vi "Manual Assembly old.vi"() -> ()   [LabVIEW 2021]
uses:
  Classes/Routine/Routine Enum.ctl
  Classes/Routine/TypeOfHexaboard.ctl
  Classes/Assembly/Assembly Run.lvclass
  Classes/Workspace/Fixture Enum.ctl
  Classes/Controller/Controller.lvclass
  Classes/Workspace/Fixture.lvclass
  Classes/Routine/Routine.lvclass
panel:
  in  "Submit":bool
  out "Type of Hexaboard Confirmation":T1
  in  "Type of Component":T1
  in  "Update":bool
  in  "Stage":i32(listbox)=-1
  in  "Routine":T2=enum."Dispense on Plate"
  in  "Stop":bool
  in  "Remove":bool
  in  "Add":bool
  in  "Go":bool
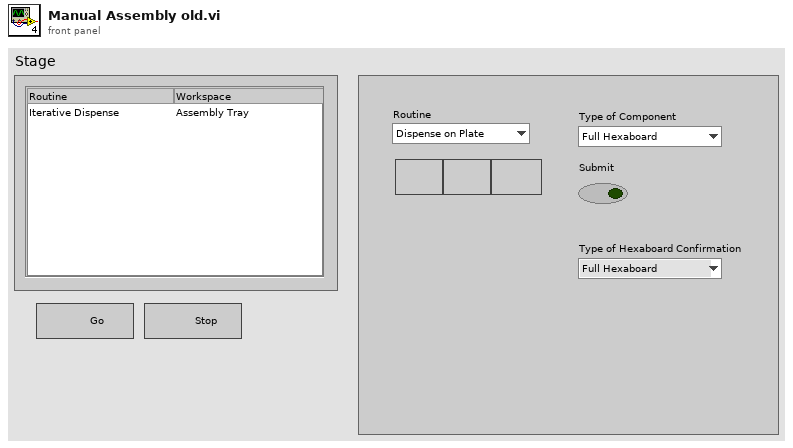
[diagram p1: front panel]
types:
  T1 = typedef "Routine.lvclass/TypeOfHexaboard.ctl" = enum16{"Full Hexaboard", "Right Partial PCB", "Right Partial Sensor", "Al Dummy Right Partial Sensor"}
  T2 = typedef "Routine.lvclass/Routine Enum.ctl" = enum16{"Primary Pick Up", "Secondary Pick Up", "Put Down All", "Secure Syringe", "Release Syringe", "Dispense on Plate", "Dispense on Sensor", "Pick Up All", "Put Down Secondary", "Dispense on Kapton"}
  T3 = typedef "Fixture.lvclass/Fixture Enum.ctl" = enum16{"Assembly Tray", "Syringe Space", "Component", "Pick Up Tool", "Current Position"}
  T4 = typedef "Controller.lvclass/Controllers.ctl" = cluster{"I-O.lvclass":refnum<class "I-O.lvclass">, "Gantry":refnum<k24>, "Dispenser":refnum<visa-resource-name>}
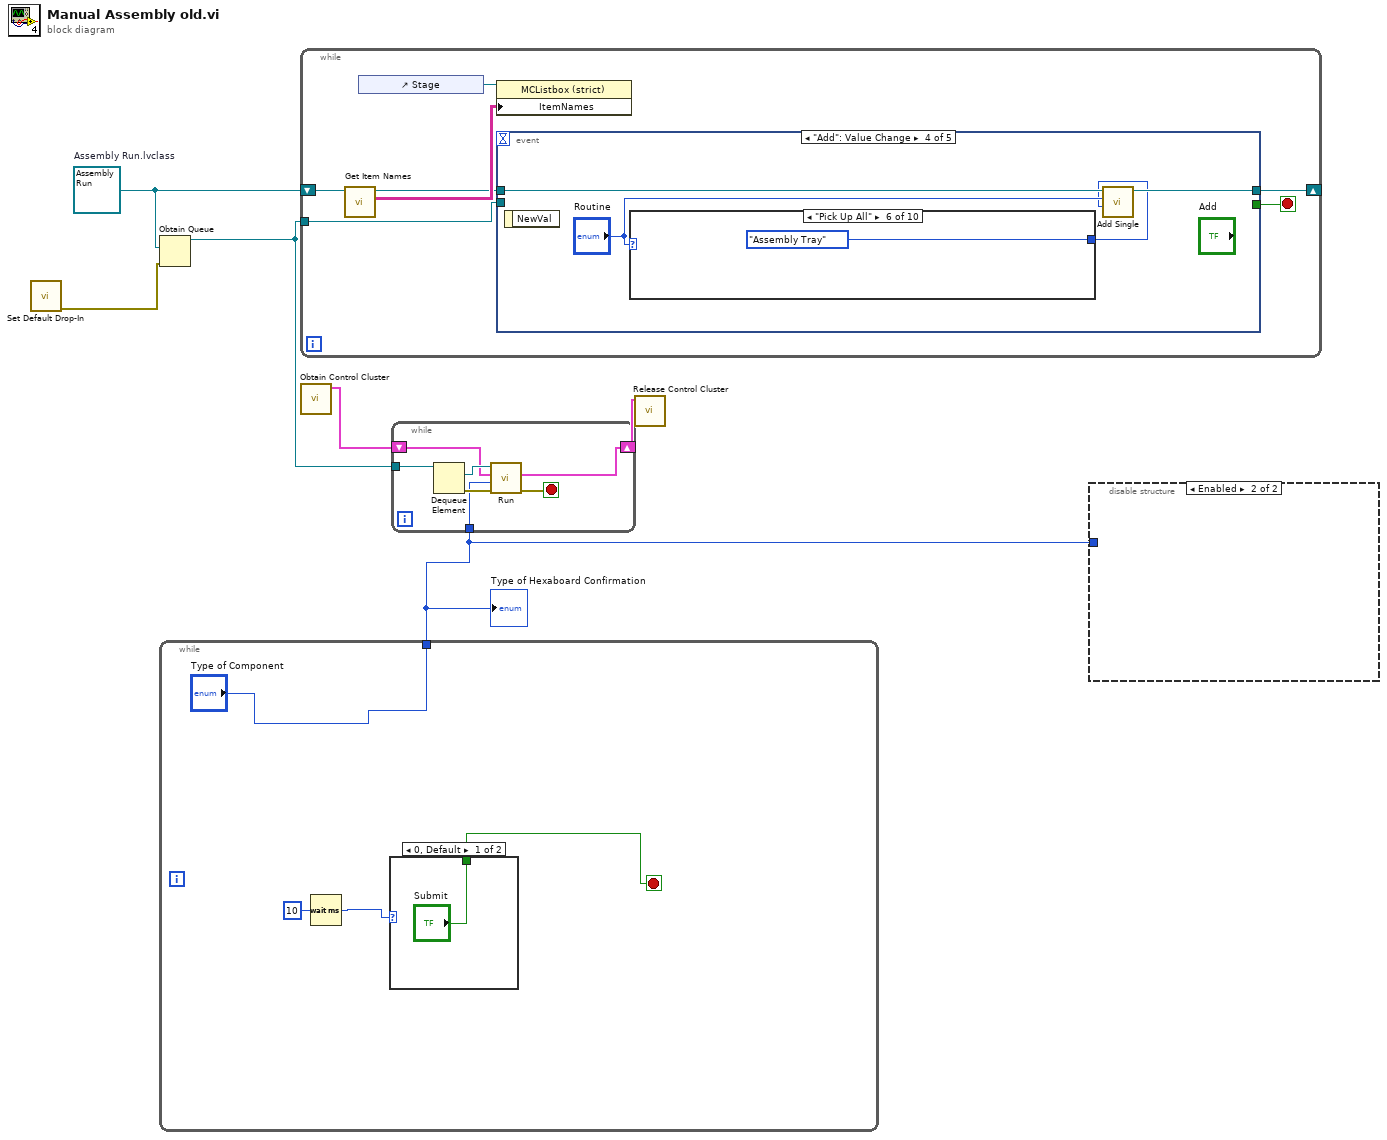
[diagram p0: block diagram]
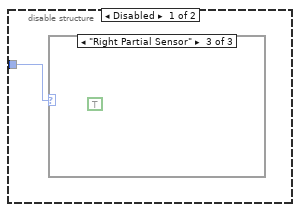
[diagram p2: hidden frame]
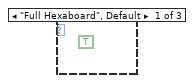
[diagram p3: hidden frame]
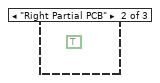
[diagram p4: hidden frame]
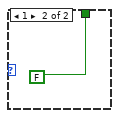
[diagram p5: hidden frame]
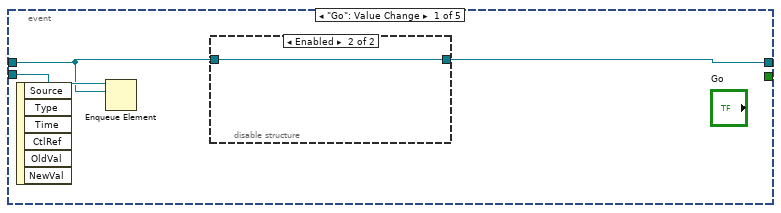
[diagram p6: hidden frame]
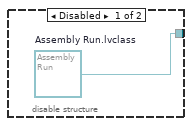
[diagram p7: hidden frame]
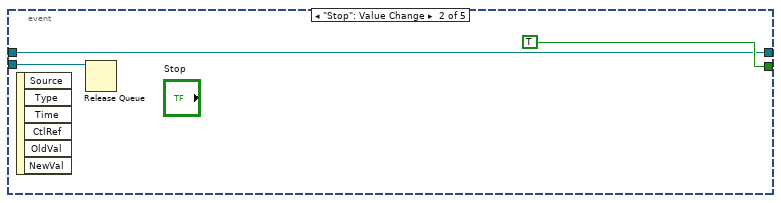
[diagram p8: hidden frame]
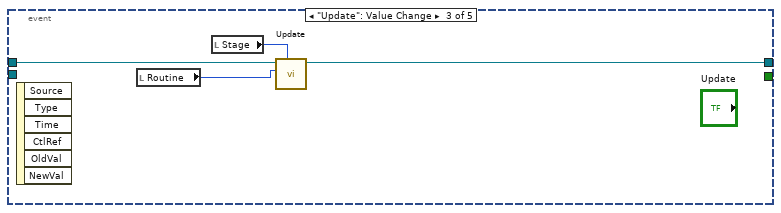
[diagram p9: hidden frame]
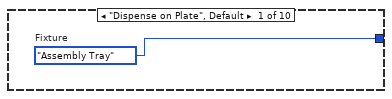
[diagram p10: hidden frame]
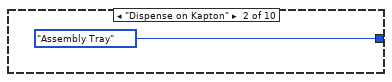
[diagram p11: hidden frame]
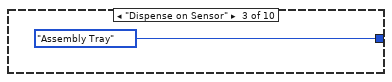
[diagram p12: hidden frame]
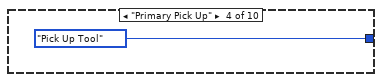
[diagram p13: hidden frame]
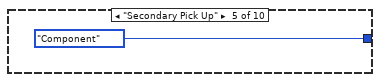
[diagram p14: hidden frame]
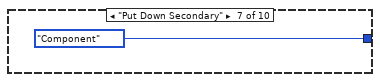
[diagram p15: hidden frame]
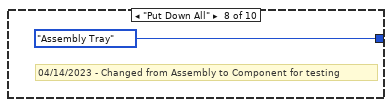
[diagram p16: hidden frame]
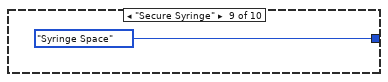
[diagram p17: hidden frame]
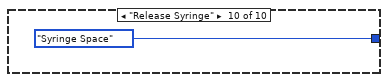
[diagram p18: hidden frame]
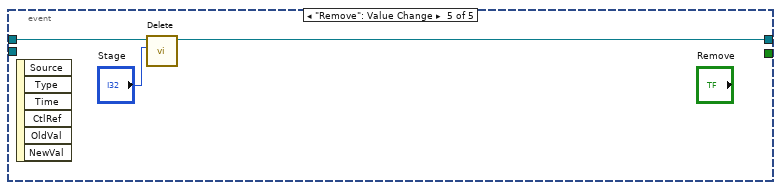
[diagram p19: hidden frame]
diagram:
  w2 = refnum<class "Assembly Run.lvclass"> refnum  # Assembly Run.lvclass
  n1 = call "Set Default Drop-In.vi"() -> ("error out"=w4:errorcluster)  [unwired: 11 in]
  n2 = Obtain Queue(element data type=w2, error in (no error)=w4) -> (queue out=w6:refnum<queue>)  [unwired: 3 in, 2 out]
  n3 = while {
    tunnel: ["Type of Component"] -> w1
    stop <- w9 stop-if-true
    n4 = Wait (ms)(milliseconds to wait=u32 10) -> (millisecond timer value=w7:u32)
    n5 = case shown="0, Default" w7 {
      tunnel: ["Submit" FALSE] -> w9
      frame 0, Default {
      }
      frame 1 {
      }
    }
  }
  "Type of Hexaboard Confirmation" <- w1
  n6 = while {
    shift-right: [w13] -> _
    shift-left: w2 -> [w15]
    tunnel: w6 -> [w18]
    stop <- w19 stop-if-true
    n7 = call "Get Item Names.vi"("Assembly Run in"=w15) -> ("Item names"=w17:string[][], "Assembly Run out"=w14:refnum<class "Assembly Run.lvclass">)  [unwired: 8 in, 1 out]
    n8 = control-ref of="Stage"() -> (w16:refnum<vi>)
    n9 = property class="MCListbox (strict)"(reference=w16, "ItemNames"=w17) -> ()  [unwired: 1 in, 2 out]
    n10 = event shown="[3] \"Add\": Value Change" {
      selector: _ -> [_ _ _ _ _]
      dyn-events: _ -> [_ _ _ _ _]
      timeout: _ -> [_ _ _ _ _]
      tunnel: [_ TRUE _ _ _] -> w19
      tunnel: w14 -> [w20 w26 w31 w35 w48]
      tunnel: [w21 w26 w30 w34 w47] -> w13
      tunnel: w18 -> [w22 w25 _ _ _]
      event "Go": Value Change {
        n11 = event-data() -> ()  [unwired: 1 in, 6 out]
        n12 = Enqueue Element(queue=w22, element=w20) -> ()  [unwired: 2 in, 3 out]
        n13 = disable-structure shown="Enabled" {
          disable-tunnel: [w23 w24] -> w21
          disable-tunnel: w20 -> [_ w24]
          frame Disabled {
            w23 = refnum<class "Assembly Run.lvclass"> refnum  # Assembly Run.lvclass
          }
          frame Enabled {
          }
        }
      }
      event "Stop": Value Change {
        n14 = event-data() -> ()  [unwired: 1 in, 6 out]
        n15 = Release Queue(queue=w25) -> ()  [unwired: 2 in, 3 out]
      }
      event "Update": Value Change {
        n16 = event-data() -> ()  [unwired: 1 in, 6 out]
        n17 = local read "Routine"() -> (w29:T2)
        n18 = local read "Stage"() -> (w28:i32)
        n19 = call "Update.vi"("Row"=w28, "Routine"=w29, "Assembly Run in"=w31) -> ("Assembly Run out"=w30:refnum<class "Assembly Run.lvclass">)  [unwired: 7 in, 1 out]
      }
      event "Add": Value Change {
        n20 = event-data() -> ()  [unwired: 1 in, 1 out]
        n21 = case shown="\"Pick Up All\"" "Routine" {
          tunnel: [w36 Fixture_Enum."Assembly Tray" ("Fixture") Fixture_Enum."Assembly Tray" ("Fixture") Fixture_Enum."Pick Up Tool" ("Fixture") Fixture_Enum."Component" ("Fixture") Fixture_Enum."Assembly Tray" ("Fixture") Fixture_Enum."Component" ("Fixture") Fixture_Enum."Assembly Tray" ("Fixture") Fixture_Enum."Syringe Space" ("Fixture") Fixture_Enum."Syringe Space" ("Fixture")] -> w32
          frame "Dispense on Plate", Default {
            w36 = Fixture_Enum."Assembly Tray"  # Fixture
          }
          frame "Dispense on Kapton" {
          }
          frame "Dispense on Sensor" {
          }
          frame "Primary Pick Up" {
          }
          frame "Secondary Pick Up" {
          }
          frame "Pick Up All" {
          }
          frame "Put Down Secondary" {
          }
          frame "Put Down All" {
            # "04/14/2023 - Changed from Assembly to Component for testing"
          }
          frame "Secure Syringe" {
          }
          frame "Release Syringe" {
          }
        }
        n22 = call-dynamic "Add Single.vi"("Fixture"=w32, "Routine"="Routine", "UI in"=w35) -> ("UI out"=w34:refnum<class "Assembly Run.lvclass">)  [unwired: 6 in, 1 out]
      }
      event "Remove": Value Change {
        n23 = event-data() -> ()  [unwired: 1 in, 6 out]
        n24 = call "Delete.vi"("Index"="Stage", "Assembly In"=w48) -> ("Assembly Out"=w47:refnum<class "Assembly Run.lvclass">)  [unwired: 8 in, 1 out]
      }
    }
  }
  n25 = call "Obtain Control Cluster.vi"() -> ("Control Out"=w3:T4)  [unwired: 11 in]
  n26 = while {
    tunnel: w6 -> [w55]
    shift-right: [w50] -> w5
    shift-left: w3 -> [w51]
    tunnel: w1 -> [w49]
    stop <- w52 stop-if-true
    n27 = Dequeue Element(queue=w55) -> (element=w54:refnum<class "Assembly Run.lvclass">, error out=w53:errorcluster)  [unwired: 2 in, 2 out]
    n28 = call-dynamic "Run.vi"("error in (no error)"=w53, "Type of Hexaboard"=w49, "Control In"=w51, "Assembly In"=w54) -> ("error out"=w52:errorcluster, "Control Out"=w50:T4)  [unwired: 5 in, 1 out]
  }
  n29 = call "Release Control Cluster.vi"("output cluster"=w5) -> ()  [unwired: 11 in]
  n30 = disable-structure shown="Enabled" {
    disable-tunnel: w1 -> [w56 _]
    frame Disabled {
      n31 = case shown="\"Right Partial Sensor\"" w56 {
        frame "Full Hexaboard", Default {
          w57 = TRUE
        }
        frame "Right Partial PCB" {
          w58 = TRUE
        }
        frame "Right Partial Sensor" {
          w59 = TRUE
        }
      }
    }
    frame Enabled {
    }
  }
